vi "ABR3-Averager.vi"(0 "Runtime":T27={"Ceiling"=0.0, "Threshold"=0.0, "Crossed?"=FALSE, "Step"=0, "Stop"=0, "Avgs"=0, "Level"=0.0, "AI Npts"=0, "Doubled?"=FALSE, "Gain"=0.0, "NWindowPts"=0, "dt"=0.0, "Cal"=path "", "Freq"=0.0, "AO Channels"=[], "AltPol"=FALSE, "AO Npts"=0, "AO Fs"=0.0, "Start"=0, "Stop max"=0, "Ear"=enum."Right", "Waveform"=enum."TONE PIP", "RepRate"=0.0, "CAP or ABR"=1, "LMasker"=0.0, "SeqVar"=enum."Signal Level", "Reps/buffer"=0, "Avg Mode"=enum."Neural/CM", "Wav"=path "", "Order"=enum."Sequential", "Levels"=[], "ControlVal"=0.0, "innerIndex"=0, "indexStep"=0} {"CAP or ABR" items=["CAP", "ABR"]}, 2 "Abort":refnum<vi>, 7 "StimChans":T1 {"Filter"."Stages"."IIR Filter"."Forward Coefficients" format="%.4f"; "Filter"."Stages"."IIR Filter"."Reverse Coefficients" format="%.4f"}, 9 "Output Scaling":enum16{"Volts", "mV", "uV"}(ring)=enum."uV", 11 "error in (no error)":errorcluster, 12 "Remove DC Offset":bool=TRUE) -> (4 "Neural (uV)":dbl[](array[numeric])=[1.4395282511290837, 1.532755910405911, 1.474410329802132, 1.2597141561756957, 0.9001139821787747, 0.4235794582247189, -0.1276333716652575, -0.6998551074240021, -1.2340253166383555, -1.6719709249654355, -1.9620685245277936, -2.0664055181998617, -1.9647336236375028, -1.6568425026802076, -1.1650092311107514, -0.532397946197658, 0.18204236523367556, 0.906952954377487, 1.568756269865719, 2.0968412700840853, 2.432608440857153, 2.535322639805393, 2.3877606906196944, 1.9984937834608272, 1.4008932321747913, 0.6517150331153516, -0.17654328788016557, -1.0008408901491515, -1.7371580487858334, -2.3098045051007574, -2.65880868149595, -2.7463184287015, -2.5615615674647567, -2.121076834648578, -1.4686197069452032, -0.6693878326519646, 0.1969045084035855, 1.0449419706065644, 1.7920868586870562, 2.3650781681900184, 2.708422476925283, 2.788258951221298, 2.5965134974653075, 2.1522809221634867, 1.499118892634998, 0.7006198878547872, -0.1655836933809833, -1.014234830616595, -1.7625943927765395, -2.3380277004402488, -2.6840320769034283, -2.7664930928624387, -2.577696725613432, -2.1357488319848748, -1.4844911055883332, -0.6869176095510444, 0.17875347261089547, 1.0279345576657934, 1.7780792466594524, 2.355328107270133, 2.7038276454865047, 2.789379765791016, 2.60328656101914, 2.1640114189129878, 1.5144932790531567, 0.7183829551330373, -0.14731347632345962, -0.9972781324467478, -1.7485157781425051, -2.3281762074883967, -2.6794144228663423, -2.767570799346762, -2.5843785020013836, -2.1474007209849293, -1.4999111371554372, -0.7047973229346518, 0.1603615387991024, 1.0107597841892353, 1.7639270959139701, 2.3453802559937347, 2.6991542049437, 2.7904042207387056, 2.6098719770818493, 2.175698807779738, 1.5300274194957273, 0.7360268414650899, -0.128827718950226, -0.97999939173869, -1.7344067345971401, -2.3181269242110836, -2.6746496937413387, -2.768354355340884, -2.590961383132333, -2.159006966335281, -1.5152474886200955, -0.7225629269268649, 0.14208878618494694, 0.9936458695053323, 1.7493844364731472, 2.3354146545365095, 2.6944680855781407, 2.7912917435799787, 2.6162798887646694, 2.1871579771640977, 1.5453764489455355, 0.7535160460710334, -0.11053721586306206, -0.962852511425284, -1.7199756482361281, -2.308184143825026, -2.6697759261858742, -2.7692494856355405, -2.597356616772928, -2.1703317409173235, -1.5306421632430864, -0.7401205980371353, 0.12379574745708481, 0.9764888470355151, 1.7351688921529747, 2.3253704442717336, 2.6894371003402995, 2.791945974715928, 2.6226878005953473, 2.1984294994708335, 1.560659548702068, 0.7711371109548816, -0.09225432013500647, -0.9458070622432678, -1.705684029790087, -2.297977642892851, -2.6647373329909874, -2.7699873975748868, -2.603721421193753, -2.181846698979479, -1.5459100496436555, -0.75789888139616, 0.10526181069266684, 0.9592126436638952, 1.7207175213235073, 2.3148342936501165, 2.6843224344912207, 2.792615420540496, 2.628991745616928, 2.209772023817738, 1.575752465912369, 0.7890193603861616, -0.07390549445381299, -0.9283153177772733, -1.691212371809544, -2.2875175645807033, -2.6595694152244445, -2.770578234287441, -2.609946757906796, -2.193143580619579, -1.5610410047193342, -0.775284120672885, 0.08693073548743217, 0.9417944374520653, 1.7060962540767397, 2.304544113599402, 2.6792686273907975, 2.793145398476443, 2.6352703329820977, 2.220942115663773, 1.5908428477332726, 0.8064705291851398, -0.05570374342245042, -0.9110492571901601, -1.676634211761152, -2.2771462387137853, -2.6543583892194644, -2.77099917377202, -2.616113771792062, -2.204300994909238, -1.5763063561495347, -0.7928925079755119, 0.06860980337863325, 0.9246779881956217, 1.6914268075380636, 2.294053607483168, 2.6740778883452796, 2.7935206938641066, 2.6413714159532464, 2.232084314306749, 1.6060422681610205, 0.8241625963892981, -0.03717487820180634, -0.8937806611422894, -1.6619926577887165, -2.2666506600838408, -2.6490991835183375, -2.771371933418275, -2.6220931381771617, -2.215283440936453, -1.5912902371939535, -0.8106302198319645, 0.05024322743833475, 0.907150744453164, 1.676990652486208, 2.2835986025019612, 2.6686487861421813, 2.7937818791869247, 2.647264565187043, 2.243013508077417, 1.6209424678155986, 0.8417912696118693, -0.018957912612517995, -0.8762762387543624, -1.6472801025639217, -2.2559927920535903, -2.6437131889822236, -2.771732014155341, -2.627943179941323, -2.226303923886866, -1.60628172595746, -0.8280357460850919, 0.031891866119443904, 0.8898288983823229, 1.6621284879701426, 2.273057381400807, 2.662991463967972, 2.7940456002231904, 2.653058819196084, 2.253805770232825, 1.6358578824782266, 0.8590167556607577, -0.0005380855097547682, -0.8589315701916806, -1.6324483663924145, -2.2454338195540005, -2.63805333037468, -2.771828373804143, -2.633742506225171, -2.2371874752419902, -1.6212554647154789, -0.845656813087822, 0.013472039033399833, 0.8726896280383284, 1.6471598213917418, 2.2621789023862293, 2.657415286783958, 2.794157174537408, 2.6585893522697233, 2.2648110378220814, 1.650829084530336, 0.8768051829424925, 0.017838633505439176, -0.8413891118434587, -1.6174644842500803, -2.234560411108988, -2.6323605067511378, -2.7718765536431547, -2.639458151899738, -2.248114135072439, -1.6360364851212237, -0.8631434845611444, -0.00492496613723117, 0.8549062723626905, 1.6324700901986882, 2.251280137430886, 2.6516717483009025, 2.7940684222685657, 2.664284711061999, 2.275598228985624, 1.6655999609317433, 0.8940458841581485, 0.03615956559409267, -0.8238770830261509, -1.6026809285518098, -2.223684467145914, -2.6265130006914403, -2.7716102967650222, -2.644950649097256, -2.2585792839095884, -1.6507110034704318, -0.8803157208139684, -0.023197718633086662, 0.8375489263325268, 1.6173619569017978, 2.2404016589553764, 2.645727883422537, 2.7938047012037854, 2.669830459010278, 2.286111556607921, 1.6802770141117271, 0.9112536206390183, 0.054675751908509915, -0.8063447683355018, -1.5876716894773257, -2.2126056614032725, -2.6205310984515395, -2.771377004987947, -2.6503746803828574, -2.26918643648586, -1.6654844173387813, -0.8979088952371275, -0.04167840421967746, 0.8198315012253321, 1.6024161134418988, 2.229322854486931, 2.639796697528131, 2.7935866241444525, 2.675234203426622, 2.296594455191442, 1.6950199977826657, 0.9287935433005925, 0.07293075400881417, -0.7887389165905049, -1.5725052328839124, -2.2015420706085287, -2.614508623853641, -2.7710194600020954, -2.6556567081065747, -2.2796870867417764, -1.6801538649249124, -0.9152256709988795, -0.05998665753082091, 0.802261151042639, 1.5873079809104267, 2.218411411520159, 2.6337640806194615, 2.7930820040137405, 2.680465514967574, 2.307072282498074, 1.70971987368572, 0.9460393169109486, 0.09130747304302385, -0.7710519204811589, -1.5574199214201694, -2.1904429792523774, -2.6085013640321106, -2.770519911348151, -2.6609463432756186, -2.29005334112161, -1.6946305941277193, -0.9324156585420217, -0.07840394894946831, 0.7847846246058203, 1.572093346330642, 2.20700042102332, 2.6275083153116934, 2.7925469545091675, 2.685757685287872, 2.317400499277337, 1.7240393840276242, 0.9633129842890915, 0.10968419209879166, -0.753651466650922, -1.5422357152114121, -2.1789914153566126, -2.6022532053450385, -2.7699392177555886, -2.665908862976646, -2.300290271169476, -1.7091681822925784, -0.9498921884640046, -0.09663866502852804, 0.7669708410226813, 1.55699535766433, 2.1958100433093706, 2.6213565169854682, 2.7918318646607405, 2.690595951286384, 2.327591784368511, 1.7385769712468833, 0.9806018665855719, 0.12802794618370078, -0.7359061483634411, -1.5270160085834796, -2.1676793194380464, -2.5960050467862326, -2.769203841576933, -2.670929705707365, -2.3104764859072207, -1.7235891252756244, -0.9670162466031, -0.11484295192375675, 0.7493421688916414, 1.5416869002770077, 2.184388910315485, 2.614849709831871, 2.7910026647306077, 2.695581292511742, 2.3377298184180635, 1.7530892011204837, 0.9976042071355885, 0.14649088145417494, -0.7183129765330382, -1.511601047868935, -2.1561973268370647, -2.589450059108852, -2.768212351653958, -2.6758161521845514, -2.320769203572741, -1.7376753465564172, -0.9841326977485383, -0.13324249309905548, 0.7320000389875209, 1.526378443274855, 2.172851131977019, 2.608287115690693, 2.7900568189398456, 2.7003485568099435, 2.3478044583237763, 1.767177957231152, 1.014984377778882, 0.1648346356155949, -0.7006411960887469, -1.4962139810501114, -2.1447127987785337, -2.582753067945189, -2.76718028921617, -2.6804997364251566, -2.3305851954349137, -1.7520278244533696, -1.0014063669930806, -0.15151271010604112, 0.714077218032654, 1.510943198040489, 2.161211922902419, 2.6014988373813863, 2.7890627933674765, 2.7049180304571885, 2.3577624527603387, 1.7815025406516098, 1.032047577434772, 0.1830313152130599, -0.6827285177541538, -1.480864951204245, -2.133030480539171, -2.575929288016269, -2.7661456910403874, -2.6850666748634477, -2.3403682224641917, -1.7660962960808266, -1.0182641701842496, -0.17005425448429284, 0.6962938646504973, 1.4952518401973722, 2.149516927099661, 2.5947587389858833, 2.7878380118160977, 2.7093911444998424, 2.367395868027308, 1.7957307650661247, 1.0489358092347998, 0.20144860678364765, -0.6650212370259554, -1.4651786640447881, -2.1212391242885063, -2.5691460806573256, -2.7648575148560206, -2.6895372537110442, -2.350250145047671, -1.7802357697758513, -1.0355834839660625, -0.1882610774014398, 0.6784192237848757, 1.4798597038465398, 2.13772810790351, 2.5878386004844325, 2.786491512905318, 2.713983440269239, 2.3771966448057107, 1.8096546970626046, 1.0661891923214208, 0.21971375226454914, -0.6470933445595164, -1.4495988797039707, -2.109404660144406, -2.5622918716404395, -2.7635591955570358, -2.694017975789843, -2.360066137666051, -1.7942104185697303, -1.0523804293216747, -0.2065490450127634, 0.6605800839202034, 1.4642393484020582, 2.125820107628723, 2.581037643661518, 2.7851830506465243, 2.718418517778739, 2.386999957583907, 1.8236217375547858, 1.0830850320699636, 0.23812597242670458, -0.6294215650763136, -1.4339404868196217, -2.0975169450698448, -2.5552829802913215, -2.762141694617366, -2.6982704777527546, -2.3694611915644925, -1.808202818153744, -1.069230626194157, -0.22486490617253674, 0.6428804116000764, 1.4482741283453793, 2.1139400011792007, 2.5738537845377714, 2.783613403096724, 2.722622839463714, 2.3965015131897376, 1.8375456702847826, 1.0999960867726546, 0.25627193689684197, -0.6113973138242079, -1.418208556934832, -2.0855049773296264, -2.5479900818666787, -2.7605187955318686, -2.702451977990576, -2.3789576767500487, -1.8221445026495653, -1.0862608631352142, -0.2431351235786486, 0.6248358748193603, 1.4326968817766805, 2.101839282613086, 2.56670289062944, 2.7819702179752674, 2.7267155868816295, 2.4057063831215246, 1.851363100909952, 1.1170719669011222, 0.27440015106205384, -0.593423778195461, -1.4024791632205018, -2.073292683680086, -2.5407986147622528, -2.7587970010102, -2.7063367920534986, -2.388028151619793, -1.835832610156751, -1.1029538428928658, -0.2616411676260088, 0.6069206624947833, 1.4169167738274846, 2.08950527309283, 2.559318705298538, 2.780210386993262, 2.730519255576555, 2.4150177558892056, 1.8650714936261625, 1.133648300526371, 0.29293915993025077, -0.5757063555185494, -1.3867066617596802, -2.061095604988597, -2.533401749733742, -2.757019419340479, -2.710231749269889, -2.397451099724693, -1.8495384684521923, -1.1197812188493002, -0.27975416754395616, 0.5890384153766166, 1.4007968728445, 2.0774045552023517, 2.551987771452443, 2.7783694110848027, 2.734388854527701, 2.4244533819758685, 1.8788052444530907, 1.1506151431865264, 0.31097355081361083, -0.5577201414662862, -1.3708251224930792, -2.0489365632824286, -2.525982062894162, -2.7550288322114613, -2.7139390588641694, -2.406623006120719, -1.8632595417744564, -1.136639024418934, -0.2980674933467866, 0.5710369872817437, 1.3851942696638073, 2.064999544634335, 2.544524977320814, 2.7763281086137757, 2.738068270089232, 2.433569500401233, 1.892191594643508, 1.1673131944801958, 0.32944662987850254, -0.539815072249307, -1.3548421527325196, -2.0364985866595875, -2.5183747286105334, -2.7528379184684173, -2.7176210106849936, -2.415554013900312, -1.8766737868174372, -1.1531697158764533, -0.3163022104208217, 0.5531648836200865, 1.3692366588161557, 2.052647785705688, 2.5367097102202263, 2.77426651989102, 2.7416995059391827, 2.4423990761528023, 1.9056109102562346, 1.1839833526370318, 0.34755962981494204, -0.5217832147506022, -1.338732394775463, -2.023999751783519, -2.5104504222139727, -2.7506825056572644, -2.721054456174375, -2.424416555892335, -1.8901260688365098, -1.1699336986288993, -0.3344278895390942, 0.5350417389593082, 1.3529417907182757, 2.0401895245525083, 2.529061804623173, 2.772067999116759, 2.7450365913761954, 2.4512083659474833, 1.9190378335383393, 1.2006687257661814, 0.365713202171782, -0.5036828916702697, -1.3227266038327146, -2.0114578090763104, -2.5027771580438016, -2.748483984603527, -2.7245234025946865, -2.4334692813996686, -1.903461705622813, -1.1865404639345887, -0.3528020741843035, 0.5170656691051284, 1.3369486798092405, 2.0276729409547323, 2.521213572754994, 2.7697046526819635, 2.7485004658019165, 2.460121622798475, 1.9324799718506473, 1.2171512375589537, 0.38406456465418054, -0.4856687849437102, -1.3065788100683984, -1.9988550081260086, -2.4948655309081023, -2.746059779182957, -2.727895989452707, -2.442057959828062, -1.9164702278679644, -1.2030914426382415, -0.37094296818746797, 0.49907945634375267, 1.3208211733750277, 2.014940816812523, 2.5132715172726376, 2.76717901640693, 2.751888266947193, 2.468766087491162, 1.9457091054933713, 1.2335602123332297, 0.40214713571509625, -0.4676597499372556, -1.2902712630602917, -1.985978343860765, -2.4868550085978316, -2.743544285699133, -2.731103750647599, -2.4506998897994006, -1.9297551499079513, -1.219604385136538, -0.38908386233475983, 0.48082191641692823, 1.304569414505728, 2.002041331921324, 2.505131671278596, 2.7645316627102106, 2.7550148828155105, 2.477446053212338, 1.958712555602921, 1.2502278361276218, 0.4204579261486709, -0.44944531777965124, -1.2741209342720257, -1.9731549312156869, -2.478715161777337, -2.7408943959175667, -2.734202473365503, -2.459235317300394, -1.9430705016025347, -1.2360082898295168, -0.4072678647114303, 0.4628382397472022, 1.288360764108287, 1.989233135263758, 2.4968777155193824, 2.761775270529009, 2.7580121739827734, 2.485826797431994, 1.97198226235536, 1.2663223759828894, 0.43853542594029116, -0.43136021003728786, -1.2578260668801813, -1.960260517237996, -2.4704257042637585, -2.7379883923770554, -2.737154120869973, -2.467550132340703, -1.9560105590457155, -1.2523589436955342, -0.4252895780008659, 0.44466438052441326, 1.2718326068925097, 1.9761840403993531, 2.4885045784086737, 2.759072129737366, 2.760989178932014, 2.494022430080994, 1.9849907847186021, 1.2828632119346168, 0.4567244997294825, -0.4132472089942173, -1.2413613031742499, -1.947297637710777, -2.4619130985201534, -2.7350925320090744, -2.739849654637991, -2.476001879577561, -1.9688136850221156, -1.2686107028535771, -0.4434634376195193, 0.4264119125985013, 1.2554895613448314, 1.9632008760101387, 2.48018215700205, 2.7561585192983045, 2.763661890395179, 2.502398103099653, 1.9977736235210932, 1.2992569735137212, 0.4749059663618254, -0.395189995035824, -1.2250740438404228, -1.934329686984774, -2.453550103807855, -2.7322296367830616, -2.7425781536119915, -2.4840910107416825, -1.9817917797900413, -1.284875141230547, -0.4615840462493072, 0.4082659471272895, 1.2391414446079814, 1.9500833159444133, 2.4717202680398254, 2.7529735805129256, 2.7663067082870416, 2.510558235239559, 2.0106705725154517, 1.3153160136362303, 0.4930316462238931, -0.3771048877654994, -1.208616888188332, -1.920923047663721, -2.4450400342361003, -2.7290878058482697, -2.745157041573262, -2.492147177009889, -1.9945162974540873, -1.301152258848653, -0.47960068850441295, 0.39000080063122333, 1.2226335746387296, 1.9368009309343408, 2.463002265760695, 2.7496821389891775, 2.768870381247518, 2.518581435549004, 2.02342551848756, 1.3316032735468908, 0.511101539322759, -0.3587104167783139, -1.1919213704095126, -1.9077015202389411, -2.4362789228363164, -2.7257405767933123, -2.747662391940525, -2.500122198520436, -2.0072002430902764, -1.317371054098585, -0.4977187617199302, 0.3719283727317753, 1.2061890992963278, 1.92351347472132, 2.4542969425528365, 2.7464591635474354, 2.7712387992446943, 2.5263916307111822, 2.035972531296324, 1.3478296753155836, 0.5291131098931647, -0.3406329171012239, -1.175489573194469, -1.8944647785399493, -2.4275330263440256, -2.722355311077759, -2.7500155955379855, -2.5078842148977607, -2.01982840201712, -1.3333464156500179, -0.5157607620370909, 0.3536733695635592, 1.1895113333591902, 1.9102589839359723, 2.4453329702870823, 2.7429597881868357, 2.773505786060023, 2.5340978591650125, 2.048481507809941, 1.363881109223582, 0.5471196090969712, -0.3223271983176138, -1.1588726650470516, -1.8813041104226378, -2.418487908311925, -2.718848327958181, -2.7522267955200954, -2.5158668441185466, -2.03249966948883, -1.3495094246851844, -0.5338433348609879, 0.3353143999708917, 1.172732136945969, 1.8967027364091325, 2.43645267889724, 2.739242335856683, 2.775711914191574, 2.5420323077444715, 2.0609473765130346, 1.3797905402927073, 0.5651844311816042, -0.30416601851249997, -1.1420655744232873, -1.8675982512369118, -2.409445326266602, -2.7151866623603533, -2.754473496425215, -2.523481785659771, -2.044747462863247, -1.3654847869969653, -0.5517712259384716, 0.3171075766438307, 1.1561735529387842, 1.883128738844377, 2.427422776844838, 2.7356897092249115, 2.7778723983060822, 2.5494621367288666, 2.0732179908859454, 1.3958064741286889, 0.5830463918891033, -0.28589833651752683, -1.125397951564641, -1.8541383625066221, -2.40048388934014, -2.7115021747773245, -2.7564869055888566, -2.5309623311651763, -2.0569343979867307, -1.3814474708374418, -0.5697295464547676, 0.29879425111070773, 1.1393233556203597, 1.8696029213461443, 2.4182584788446406, 2.731888576306216, 2.779789447598124, 2.5569274667466364, 2.085415068122787, 1.4116601189541702, 0.6010604989617646, -0.26755965309759877, -1.1084691446454, -1.8404958984414477, -2.391294232607866, -2.7076604688784283, -2.7583912762301237, -2.538356660340975, -2.069311516582715, -1.3972351868021582, -0.5875915079333405, 0.28062039298224223, 1.1225010521159988, 1.856039067605407, 2.4088583537645163, 2.7278287939194765, 2.781622816185109, 2.56428883002743, 2.097749077525349, 1.4274503698659096, 0.6189097812081693, -0.24937311594237316, -1.091781236314106, -1.8267951119573107, -2.3819143928813644, -2.703620972281197, -2.760181536797, -2.5454390889296374, -2.0813868782604774, -1.4129544373101186, -0.6053063949823206, 0.2624008910962351, 1.1056609985605057, 1.8420137034257023, 2.39957233892674, 2.723931301453807, 2.783253322407029, 2.5713078634310507, 2.109771186958021, 1.443126511416476, 0.636819922128619, -0.23102682542586872, -1.0748245366173617, -1.8127418532700716, -2.3725548395654346, -2.6995003307628203, -2.7616294670967103, -2.5528993486569473, -2.0934039174323193, -1.4287801906321023, -0.6233788257829277, 0.24387963275702965, 1.0857754847470877, 1.8183295781965265, 2.367766091419394, 2.681223712822552, 2.729535373267443, 2.510314800597094, 2.0495693551720833, 1.3966559576513389, 0.620880074203631, -0.19861208734554114, -0.9789115461709459, -1.6430833982317077, -2.128138969482868, -2.3907033965627424, -2.411093581531485, -2.1951569867251726, -1.7721872242646255, -1.191421823477356, -0.5169145371876932, 0.1811954183282487, 0.8320260192072704, 1.3735880428904998, 1.7568776462956084, 1.9517417122730605, 1.9484832424464051, 1.7574025513572042, 1.408447296149037, 0.9447283236692902, 0.419730160344384, -0.11159716737835836, -0.5955411458827827, -0.9874063775542169, -1.2546157802529583, -1.379784004482954, -1.3610801513550121, -1.2109675481519084, -0.9550093732829174, -0.627291518489845, -0.26658338192841746, 0.08874381043064897, 0.4034150203824767, 0.6498258847102212, 0.8098786040255699, 0.8766023213339516, 0.8521169252825707, 0.7488451579968964, 0.5856734491572843, 0.3851245162283366, 0.1722999400598037, -0.030586949941910264, -0.2034909073282034, -0.33348204757844413, -0.4118829650461492, -0.43841218486660727, -0.4169443608101003, -0.3569556643837709, -0.2693575135107263, -0.16766809566460772, -0.06467783047578858, 0.028854014681161364, 0.10485101608964346, 0.15798552308759484, 0.18696429320988187, 0.1926114511761961, 0.17884729607034774, 0.1507180086533576, 0.11386567543666899, 0.07446996588255672, 0.037034405949865054, 0.005588332752696505, -0.018004463411863306, -0.03256231411188295, -0.0387064827707768, -0.037732747415657235, -0.03162407952533104, -0.0224623455792114, -0.01218994475038231, -0.002381589680865408, 0.005978841201505198, 0.012041865234115462, 0.01583284010978839, 0.017579985052400333, 0.017714380817214773, 0.01692575661235741, 0.015518404735495985, 0.014085695167122504, 0.012924312897508946, 0.01187450447036647, 0.011341992949343146, 0.011128988340931728, 0.010905840655928301, 0.010931198347405932, 0.011080808727124046, 0.011068129881385325, 0.011098559111158375, 0.011073201419680913, 0.0111061664186016, 0.01112898834093141, 0.011134059879227318, 0.01113152411007946, 0.01110109488030622, 0.011108702187749387, 0.0111010948803062, 0.011101094880306198, 0.011093487572863183, 0.011141667186670394, 0.011113773726045204, 0.011128988340931543, 0.01111630949519282, 0.011096023342010609, 0.011116309495192893, 0.011151810263261631, 0.011088416034567443, 0.011052915266498896, 0.011101094880306087, 0.011078272957976618, 0.011136595648374877, 0.011161953339852548, 0.011144202955818366, 0.011078272957976353, 0.011149274494113844, 0.011116309495192633, 0.011131524110079437, 0.011116309495192746, 0.011096023342010588, 0.011060522573941708, 0.011123916802636231, 0.011172096416443577, 0.011085880265419842, 0.011113773726045183, 0.011149274494113596, 0.011156881801556922, 0.011083344496272, 0.011136595648374917, 0.01113152411007942, 0.011098559111158392, 0.011131524110079718, 0.011139131417522815, 0.01109602334201091, 0.011101094880306387, 0.011098559111158413, 0.011118845264340491, 0.011146738724965926, 0.011106166418601711, 0.01108588026541958, 0.01112138103348841, 0.011169560647295847, 0.011136595648374976, 0.011121381033488597, 0.011134059879227056, 0.011156881801556844, 0.011101094880306481, 0.011106166418601546, 0.011098559111158526, 0.011080808727124122, 0.011134059879226929, 0.011090951803715264, 0.01110363064945423, 0.011111237956897118, 0.011123916802636193, 0.011085880265419469, 0.011144202955818068, 0.011106166418601526, 0.011149274494113806, 0.011083344496271928, 0.011108702187749538, 0.011174632185591364, 0.01113152411007914, 0.011126452571783397, 0.011134059879227469, 0.011131524110079232, 0.011156881801556712, 0.011101094880306086, 0.011103630649453947, 0.01112138103348818, 0.011149274494113865, 0.011096023342010722, 0.011154346032409002, 0.011108702187749387, 0.0111416671866706, 0.011096023342010592, 0.011172096416443424, 0.01108588026541975, 0.011108702187749725, 0.011146738724965796, 0.011174632185591418, 0.011090951803715226, 0.011103630649453853, 0.011085880265419637, 0.011128988340931522, 0.011113773726044884, 0.011083344496271814, 0.011116309495192572, 0.011156881801556882, 0.011131524110079158, 0.011106166418601847, 0.011134059879227113, 0.011111237956897379, 0.011141667186670602, 0.011070665650533561, 0.01113913141752263, 0.01115688180155677, 0.011159417570704705, 0.011088416034567308, 0.011111237956897476, 0.011128988340931633, 0.011156881801557161, 0.011057986804794747, 0.011111237956897268, 0.011113773726045037, 0.011146738724965927, 0.01112898834093173, 0.01111630949519295, 0.011146738724965927, 0.011126452571783942, 0.011085880265419939, 0.011075737188828642, 0.011123916802636025, 0.011093487572863069, 0.011078272957976221, 0.011113773726044978, 0.011108702187749502, 0.011123916802635837, 0.01106559411223724, 0.011123916802636214, 0.011093487572862956, 0.011141667186670262, 0.011073201419681085, 0.011136595648374749, 0.011108702187749687, 0.0111568818015569, 0.01108334449627153, 0.011136595648374955, 0.011075737188828552, 0.01112898834093192, 0.01112391680263614, 0.011134059879227168, 0.011098559111158281, 0.011103630649454044, 0.011131524110079682, 0.011070665650533261, 0.011134059879226983, 0.011134059879227207, 0.011103630649454117, 0.01112645257178387, 0.011085880265419769, 0.011123916802636065, 0.011144202955818368, 0.011128988340931543, 0.011088416034567476, 0.01113152411007929, 0.011108702187749649, 0.01112645257178398, 0.011098559111158226, 0.011111237956897302, 0.011121381033488201, 0.011154346032409414, 0.011073201419681065, 0.01113913141752259, 0.011098559111158564, 0.011111237956897174, 0.011174632185591045, 0.011121381033488297, 0.01108334449627164, 0.011111237956897436, 0.011121381033488427, 0.011128988340931558, 0.011101094880306351, 0.011090951803715358, 0.011146738724965966, 0.011136595648374785, 0.011164489109000314, 0.011085880265419675, 0.01114927449411377, 0.011131524110079645, 0.011187311031329954, 0.011060522573942137, 0.011136595648374954, 0.011078272957976204, 0.011139131417522534, 0.011111237956897321, 0.011136595648374936, 0.011096023342010609, 0.011126452571783962, 0.01113405987922713, 0.01112138103348858, 0.011123916802636176, 0.011146738724965665, 0.01114673872496585, 0.011085880265419316, 0.011131524110079513, 0.011131524110079265, 0.01108080872712427, 0.011126452571784037, 0.011093487572862862, 0.011101094880306236, 0.01115434603240915, 0.011113773726045316, 0.011085880265419524, 0.011068129881385532, 0.011073201419680876, 0.011134059879226907, 0.011070665650533013, 0.011136595648375104, 0.011080808727124386, 0.011164489109000409, 0.011101094880306351, 0.011088416034567741, 0.011101094880306594, 0.011083344496271796, 0.011121381033488297, 0.011164489109000426, 0.011118845264340755, 0.011116309495192784, 0.011151810263261367, 0.011116309495192952, 0.011159417570704743, 0.011113773726045089, 0.011131524110079212, 0.011111237956897476, 0.011128988340931786, 0.011113773726044846, 0.011151810263261406, 0.01114166718667013, 0.011134059879226941, 0.011080808727124197, 0.011131524110079479, 0.011088416034567219, 0.011156881801556844, 0.011078272957976525, 0.011136595648374749, 0.01109095180371519, 0.011174632185591043, 0.011098559111158243, 0.011090951803715263, 0.011121381033487974, 0.011113773726045146, 0.011116309495192836, 0.011151810263261312, 0.011035164882464619, 0.011136595648374877, 0.011101094880306184, 0.011068129881385383, 0.011093487572862937, 0.011093487572863069, 0.011090951803715322, 0.011159417570704818, 0.011154346032409059, 0.011161953339852359, 0.01112898834093173, 0.011057986804794294, 0.011083344496271812, 0.011106166418601921, 0.011093487572862916, 0.011141667186670264, 0.011126452571783905, 0.0110605225739421, 0.011126452571784112, 0.011139131417522534, 0.011101094880306216, 0.011113773726044995, 0.01111884526434055, 0.011111237956897117, 0.011083344496272095, 0.011073201419680894, 0.01114420295581794, 0.011121381033488505, 0.011098559111158526, 0.01108841603456761, 0.011090951803715453, 0.011144202955818179, 0.011134059879227075, 0.01109855911115849, 0.011103630649454063, 0.011136595648374785, 0.011128988340931635, 0.011113773726044772, 0.01109855911115849, 0.0111847752621823, 0.011090951803715152, 0.011134059879227337, 0.011146738724966004, 0.011103630649454023, 0.011139131417522685, 0.011116309495192876, 0.0111340598792273, 0.011090951803715094, 0.0111112379568974, 0.01108588026541956, 0.011101094880306275, 0.011080808727124311, 0.011078272957976299, 0.011090951803715339, 0.011108702187749593, 0.011116309495192989, 0.011134059879227338, 0.011118845264340586, 0.011113773726045223, 0.01109855911115849, 0.011101094880306145, 0.011121381033488446, 0.01114420295581833, 0.011096023342010817, 0.01109348757286305, 0.011118845264340453, 0.011088416034567497, 0.011134059879227057, 0.011136595648374822, 0.011144202955818236, 0.011108702187749425, 0.011134059879227262, 0.011126452571783832, 0.011136595648375087, 0.011085880265419373, 0.011050379497351315, 0.011083344496271927, 0.011156881801556993, 0.011118845264340548, 0.011123916802636177, 0.011121381033488484, 0.011088416034567422, 0.011101094880306164, 0.011136595648375104, 0.011126452571783792, 0.011096023342010609, 0.011149274494113695, 0.011098559111158545, 0.011065594112237538, 0.011106166418601827, 0.011108702187749576, 0.011136595648375049, 0.01106559411223739, 0.01115181026326148, 0.011161953339852922, 0.011096023342010852, 0.011057986804794334, 0.011118845264340286, 0.011096023342010836, 0.011118845264340848, 0.011101094880306332, 0.011113773726045204, 0.011136595648374823, 0.011164489109000164, 0.011103630649453855, 0.011108702187749668, 0.011103630649453532, 0.011085880265419599, 0.011139131417522964, 0.011085880265419786, 0.011088416034567554, 0.01113659564837484, 0.011134059879227151, 0.011060522573941897, 0.011123916802635856, 0.011106166418601716, 0.011118845264340625, 0.01108588026541973, 0.011108702187749465, 0.011042772189907844, 0.011161953339852699, 0.01106559411223771, 0.011098559111158528, 0.011096023342010968, 0.011149274494113844, 0.01110109488030635, 0.011111237956897453, 0.011159417570704837, 0.011090951803715263, 0.011078272957976676, 0.011080808727124006, 0.011149274494113546, 0.011123916802636195, 0.011083344496272058, 0.011118845264340567, 0.01111377372604486, 0.01115434603240902, 0.011113773726045297, 0.011121381033488467, 0.011090951803715058, 0.01111123795689697, 0.011093487572863011, 0.01115688180155739, 0.011118845264340756, 0.011090951803715058, 0.011113773726045204, 0.011057986804794107, 0.011113773726044808, 0.01111123795689755, 0.01111377372604511, 0.011098559111158677, 0.011113773726045183, 0.011088416034567197, 0.01108080872712414, 0.01109095180371515, 0.011151810263261253, 0.011111237956897342, 0.011116309495192838, 0.011103630649453853, 0.011121381033488389, 0.011118845264340737, 0.011111237956897325, 0.011068129881385457, 0.01108588026541975, 0.011103630649454065, 0.011088416034567271, 0.011098559111158188, 0.01111377372604509, 0.011139131417522347, 0.01111123795689721, 0.01115434603240932, 0.01107066565053273, 0.01113913141752272, 0.011116309495192819, 0.011164489109000107, 0.011103630649454023, 0.011093487572862843, 0.011123916802635988, 0.01109855911115849, 0.011164489109000053, 0.011116309495192912, 0.01111884526434051, 0.011123916802635763, 0.011090951803715113, 0.011136595648374839, 0.011088416034567667, 0.011085880265419654, 0.011108702187749576, 0.011151810263261537, 0.011154346032408948, 0.011088416034567554, 0.011055451035646395, 0.011118845264340399, 0.011131524110079309, 0.01110363064945404, 0.011090951803715134, 0.011093487572862784, 0.011101094880306124, 0.011151810263261366, 0.011108702187749349, 0.011182239493034738, 0.011141667186670133, 0.011151810263261572, 0.011113773726045146, 0.011144202955818328, 0.011088416034567401, 0.011106166418601394, 0.01112645257178385, 0.011154346032409135, 0.011101094880306387, 0.0110782729579762, 0.011085880265419805, 0.011121381033488354, 0.011101094880306276, 0.011083344496271928, 0.011131524110079309, 0.011088416034567687, 0.011121381033488316, 0.011113773726045259, 0.011118845264340567, 0.011123916802636288, 0.0110985591111583, 0.011088416034567573, 0.011083344496272114, 0.01109348757286303, 0.011131524110079496, 0.011063058343089962, 0.011141667186670449, 0.011131524110079422, 0.011106166418601808, 0.011108702187749444, 0.011093487572862973, 0.011139131417522796, 0.011144202955818062, 0.01113405987922732, 0.011128988340931673, 0.011078272957976223, 0.011126452571784, 0.011154346032409286, 0.011106166418601753, 0.011108702187749687, 0.011126452571784016, 0.011113773726045316, 0.011106166418601677, 0.011070665650533166, 0.011106166418601753, 0.011078272957976353, 0.011128988340931524, 0.011060522573942142, 0.011151810263261498, 0.011093487572863388, 0.01108588026541958, 0.01107320141968099, 0.011164489109000182, 0.011096023342010741, 0.011134059879227132, 0.011085880265419542, 0.011121381033488448, 0.01113405987922747, 0.011106166418601788, 0.011118845264340304, 0.011128988340931673, 0.01109095180371536, 0.011093487572863181, 0.011111237956897474, 0.011139131417522477, 0.01113405987922732, 0.011088416034567516, 0.01111630949519265, 0.011111237956897248, 0.011139131417522702, 0.011088416034567573, 0.011096023342010743, 0.01113913141752276, 0.011093487572862975, 0.011222811799398704, 0.011118845264340718, 0.011151810263261461, 0.01106052257394206, 0.011126452571783903, 0.011113773726044995, 0.011083344496271588, 0.011116309495192838, 0.011118845264340382, 0.011139131417522664, 0.011134059879226997, 0.011101094880306124, 0.011113773726045016, 0.01108080872712401, 0.011106166418601808, 0.0111315241100791, 0.01109095180371515, 0.01110109488030633, 0.01106052257394212, 0.011098559111158528, 0.011068129881385365, 0.0111112379568974, 0.011134059879227247, 0.011136595648375104, 0.011101094880306313, 0.011088416034567271, 0.011090951803715192, 0.011136595648374917, 0.011113773726045037, 0.011090951803715223, 0.011090951803715209, 0.01116956064729579, 0.011098559111158509, 0.011126452571784035, 0.011172096416443558, 0.011123916802636233, 0.011093487572862862, 0.011126452571783981, 0.011111237956897453, 0.011078272957976318, 0.011078272957976637, 0.011136595648374745, 0.011111237956897547, 0.011128988340931692, 0.011144202955818272, 0.011098559111158564, 0.011073201419681102, 0.011141667186670283, 0.011101094880306145, 0.011128988340931355, 0.011131524110079326, 0.011128988340931449, 0.011123916802636157, 0.011093487572863239, 0.01109095180371513, 0.011123916802636288, 0.011128988340931617, 0.011065594112237521, 0.011121381033488299, 0.011073201419680722, 0.01111884526434055, 0.011156881801556901, 0.011131524110079534, 0.01108588026541958, 0.011098559111158472, 0.011116309495192553, 0.011118845264340716, 0.01112645257178398, 0.01114673872496621, 0.011134059879227207, 0.01111123795689736, 0.01119745410792087, 0.011159417570704684, 0.011093487572863011, 0.011118845264340418, 0.0111112379568971, 0.01113659564837441, 0.011167024878148192, 0.01108080872712429, 0.01112391680263631, 0.011085880265419654, 0.011128988340931427, 0.011136595648374954, 0.011108702187749595, 0.011149274494113787, 0.011073201419680953, 0.011113773726044883, 0.011123916802636327, 0.011103630649453928, 0.011149274494113525, 0.011098559111158677, 0.01109602334201078, 0.011167024878147988, 0.011123916802636347, 0.011080808727124308, 0.011156881801557201, 0.011042772189907749, 0.01112138103348824, 0.011096023342010871, 0.011098559111158791, 0.01112645257178385, 0.011118845264340678, 0.011045307959055629, 0.011121381033488446, 0.011121381033488014, 0.011141667186670338, 0.01106812988138521, 0.011090951803715209, 0.011101094880306108, 0.011116309495193063, 0.011128988340931765, 0.011080808727124141, 0.011134059879227281, 0.011121381033488482, 0.011106166418601753, 0.011111237956897436, 0.011136595648374954, 0.011111237956897361, 0.011118845264340345, 0.011144202955818217, 0.01110363064945408, 0.011123916802636177, 0.011063058343089675, 0.011093487572863181, 0.01108334449627172, 0.01112645257178398, 0.011113773726045184, 0.011113773726044938, 0.011121381033488429, 0.011149274494113712, 0.011088416034567759, 0.011144202955817953, 0.011106166418601845, 0.011164489109000314, 0.011037700651612064, 0.011106166418601881, 0.011093487572863048, 0.011085880265419689, 0.011118845264340621, 0.011101094880306351, 0.011131524110079345, 0.01109095180371502, 0.011106166418601978, 0.011136595648374764, 0.011103630649453985, 0.011123916802636327, 0.01114927449411336, 0.011090951803714947], 6 "microphonic (uV)":dbl[](array[numeric]), 8 "StimChans out":T1 {"Filter"."Stages"."IIR Filter"."Forward Coefficients" format="%.4f"; "Filter"."Stages"."IIR Filter"."Reverse Coefficients" format="%.4f"}, 10 "Averaging data":cluster{i32, i32}, 15 "error out":errorcluster)   [LabVIEW 2020]
uses:
  TypeDefs/ABR3-Runtime Data.ctl
  epl-vi-lib/Utility VIs/Type Defs/Left-Right ring.ctl
  TypeDefs/ABR-Waveform Enum.ctl
  TypeDefs/ABR3-Seq Var Enum.ctl
  epl-vi-lib/Signal Synthesis VIs/Controls/Multichannel (Full)/Data.ctl
  epl-vi-lib/Signal Synthesis VIs/Controls/Stimulus Channel (Full)/Full Stimulus Channel Data.ctl
  epl-vi-lib/Signal Synthesis VIs/Controls/Waveform XCtl/Waveform Data.ctl
  epl-vi-lib/Signal Synthesis VIs/Controls/Waveform XCtl/Waveform Enum.ctl
  epl-vi-lib/Signal Synthesis VIs/Waveform VIs/Tone VIs/Tone Params.ctl
  epl-vi-lib/Signal Synthesis VIs/Waveform VIs/Pulse Train VIs/Pulse Train Params.ctl
  epl-vi-lib/Signal Synthesis VIs/Waveform VIs/Pulse Train VIs/Pulse Polarity.ctl
  epl-vi-lib/Signal Synthesis VIs/Waveform VIs/Pulse Train VIs/PT-Continuous State.ctl
  epl-vi-lib/Signal Synthesis VIs/Waveform VIs/Noise VIs/Noise Params.ctl
  epl-vi-lib/Signal Synthesis VIs/Waveform VIs/File VIs/StimFile-Params.ctl
  epl-vi-lib/Signal Synthesis VIs/Waveform VIs/FM Sweep VIs/FM Sweep Params.ctl
  epl-vi-lib/Signal Synthesis VIs/Waveform VIs/Chirp Train VIs/Chirp Train.ctl
  epl-vi-lib/Signal Synthesis VIs/Waveform VIs/Chirp Train VIs/Chirp Train Params.ctl
  epl-vi-lib/Signal Synthesis VIs/Waveform VIs/Complex Tone VIs/CT-Params.ctl
  epl-vi-lib/Signal Synthesis VIs/Waveform VIs/Complex Tone VIs/CT-Phase Enum.ctl
  epl-vi-lib/Signal Synthesis VIs/Waveform VIs/Complex Tone VIs/CT-Runtime Data.ctl
  epl-vi-lib/Signal Synthesis VIs/Waveform VIs/Moving Ripple VIs/Moving Ripple.ctl
  epl-vi-lib/Signal Synthesis VIs/Waveform VIs/Moving Ripple VIs/Moving Ripple.Params.ctl
  epl-vi-lib/Signal Synthesis VIs/Waveform VIs/Moving Ripple VIs/Moving Ripple.Data.ctl
  epl-vi-lib/Signal Synthesis VIs/Controls/Advanced Filter XCtl/Filter Data.ctl
  epl-vi-lib/Signal Synthesis VIs/Filter VIs/Filter-Bandwidth Units.ctl
  epl-vi-lib/Signal Synthesis VIs/Controls/Burst XCtl/Burst Data.ctl
  epl-vi-lib/Signal Synthesis VIs/Controls/Level XCtl/Level Data.ctl
  epl-vi-lib/Signal Synthesis VIs/Controls/Level XCtl/Level Units.ctl
  epl-vi-lib/Signal Synthesis VIs/Controls/Advanced Options XCtl/Advanced Stimulus Options.ctl
  epl-vi-lib/Signal Synthesis VIs/Modulation VIs/SAM VIs/SAM Params.ctl
  epl-vi-lib/PXI DAQ VIs/DAQ Engine VIs/PXI Globals.vi
  epl-vi-lib/Utility VIs/Conversion VIs/Create Waveform Cluster (2D).vi
  epl-vi-lib/Signal Synthesis VIs/Controls/Advanced Filter XCtl/Advanced Filter XCtl.xctl
  epl-vi-lib/Signal Synthesis VIs/Controls/Level XCtl/Level XCtl.xctl
  epl-vi-lib/Signal Synthesis VIs/Controls/Burst XCtl/Burst Control.xctl
  epl-vi-lib/Signal Synthesis VIs/Controls/Waveform XCtl/Waveform XCtl.xctl
  epl-vi-lib/Signal Synthesis VIs/Controls/Stimulus Channel (Full)/Stimulus Channel (Full).xctl
  epl-vi-lib/Signal Synthesis VIs/Controls/Multichannel (Full)/Multichannel (Full).xctl
  epl-vi-lib/Signal Synthesis VIs/Controls/Advanced Options XCtl/Advanced Stimulus Options.xctl
panel:
  out "Error":bool
  in  "Reject Override":bool
  in  "Rej Thresh µV":dbl=15.0
  out "Reject":bool
  out "Average":cluster{"offset":dbl, "dx":dbl, "Y":dbl[][]}(graph)
  out "#Aves":i32=120
  out "#Tries":i32=120
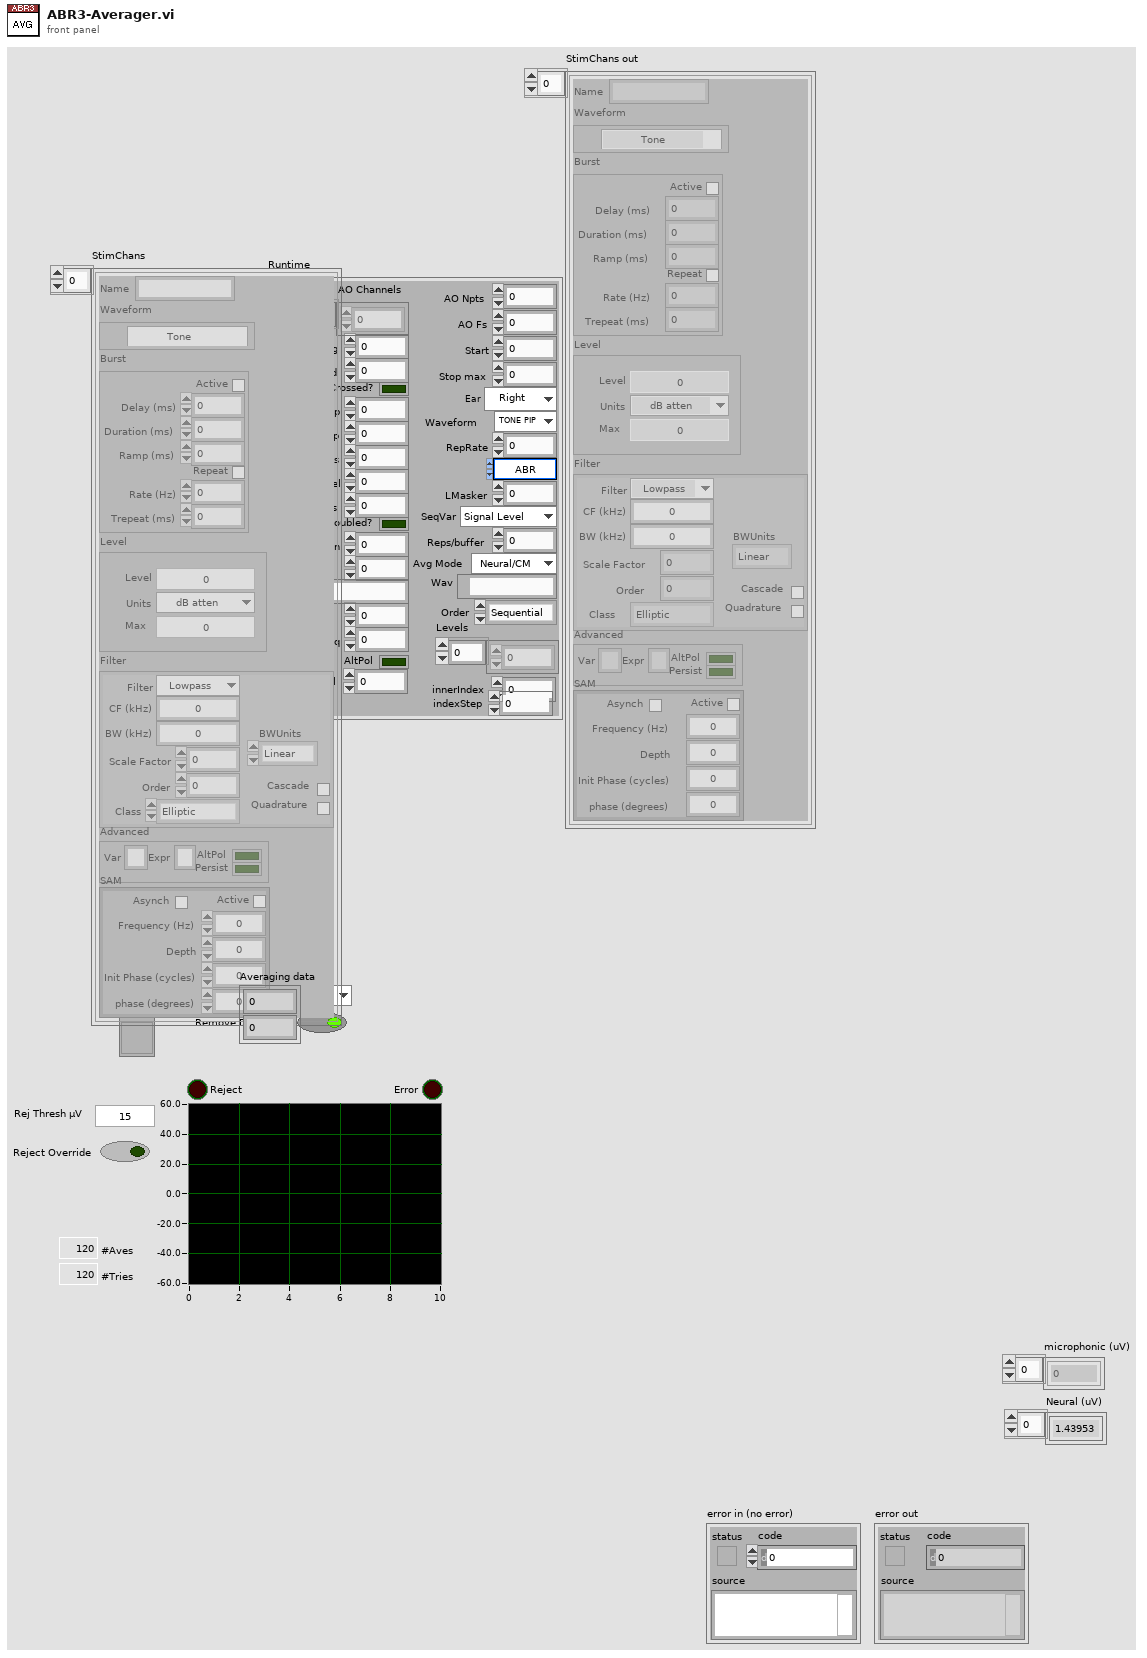
[diagram p1: front panel]
types:
  T1 = typedef "Multichannel (Full).xctl/Data.ctl" = T2[]
  T2 = typedef "Stimulus Channel (Full).xctl/Full Stimulus Channel Data.ctl" = cluster{"Waveform":T3, "Filter":T20, "Burst":T22, "Level":T23, "Name":string, "Advanced":T25, "SAM":T26}
  T3 = typedef "Waveform XCtl.xctl/Waveform Data.ctl" = cluster{"Type":T4, "Tone":T5, "Pulse Train":T6, "Noise":T9, "File":T10, "FMSweep":T11, "Chirp Train":T12, "Complex Tone":cluster{"Params":T14, "Data":T16}, "Moving Ripple":T17}
  T4 = typedef "Waveform Enum.ctl" = enum16{"OFF", "Tone", "Noise", "Pulse Train", "File", "FM Sweep", "Chirp Train", "Complex Tone", "FM Tone", "Moving Ripple"}
  T5 = typedef "Tone Params.ctl" = cluster{"Frequency (kHz)":dbl, "Last Freq":dbl, "Last Phase":dbl}
  T6 = typedef "Pulse Train Params.ctl" = cluster{"Pulse width (us)":dbl, "Pulse rate (Hz)":dbl, "Gap (ms)":dbl, "Polarity":T7, "PT State":T8, "Asynch":bool}
  T7 = typedef "Pulse Polarity.ctl" = enum16{"POS", "NEG", "POS-NEG", "NEG-POS"}
  T8 = typedef "PT-Continuous State.ctl" = cluster{"Template":dbl[], "Nperiod":i32, "Index":i32, "Pulse Rate (Hz)":dbl, "Phase (cycles)":dbl, "Noff":i32}
  T9 = typedef "Noise Params.ctl" = cluster{"InvFilt":bool, "Noise":dbl[], "CurPt":i32, "Aweight":bool, "Seed":i32, "afile":path}
  T10 = typedef "StimFile-Params.ctl" = cluster{"Filename":path, "Signal":dbl[], "Channel":i32, "stream":bool, "offset":i32, "nreps":i32, "loops":i32, "Randomize":bool, "order":i32[], "Seed":i32, "Tokens":i32}
  T11 = typedef "FM Sweep Params.ctl" = cluster{"Rate (oct/s)":dbl, "Fmin (Hz)":dbl, "Fmax (Hz)":dbl, "Ramp (ms)":dbl, "Linear":bool}
  T12 = typedef "Chirp Train.ctl" = cluster{"Params":T13, "Data":cluster{"WF":dbl[]}}
  T13 = typedef "Chirp Train Params.ctl" = cluster{"Fmin (kHz)":dbl, "Fmax (kHz)":dbl, "Compensate":bool, "Duration (ms)":dbl}
  T14 = typedef "CT-Params.ctl" = cluster{"F0 (Hz)":dbl, "Band":cluster{"Flow (Hz)":dbl, "Fhigh (Hz)":dbl}, "Phase":T15, "Min F0 (Hz)":dbl, "Max F0 (Hz)":dbl, "ContinRandPhase":bool, "Max peak factor":dbl, "Max mod depth":dbl, "MinHarmNum":i32, "MaxHarmNum":i32, "Level Mode":enum16{"per component", "overall rms"}, "% jitter":dbl}
  T15 = typedef "CT-Phase Enum.ctl" = enum16{"Cosine", "Random", "Alternating"}
  T16 = typedef "CT-Runtime Data.ctl" = cluster{"Ncomp":i32, "MinHarm":i32, "Phase":dbl[], "Amplitude":dbl[], "Npts/frame":i32, "Last F0":dbl, "Fmin":dbl, "Fmax":dbl, "Lslope":dbl, "randphase":bool, "overall rms":bool, "fmult":dbl[], "jittered":bool}
  T17 = typedef "Moving Ripple.ctl" = cluster{"Params":T18, "Data":T19}
  T18 = typedef "Moving Ripple.Params.ctl" = cluster{"Fmin":dbl, "Fmax":dbl, "Density":dbl, "Velocity":dbl, "Depth":dbl, "Phase":dbl, "Comp/oct":i32}
  T19 = typedef "Moving Ripple.Data.ctl" = cluster{"Freq":dbl[], "A":dbl[], "phase":dbl[], "Phase":dbl}
  T20 = typedef "Advanced Filter XCtl.xctl/Filter Data.ctl" = cluster{"Type":enum16{"Lowpass", "Highpass", "Bandpass", "Bandstop", "OFF"}, "CF (kHz)":dbl, "BW (kHz)":dbl, "Cascade":bool, "Quadrature":bool, "Scale Factor":dbl, "Stages":cluster{"IIR Filter":cluster{"filter structure":enum32{"IIR 2nd Order", "IIR 4th Order"}, "Reverse Coefficients":dbl[], "Forward Coefficients":dbl[]}, "State":dbl[]}[], "Class":enum16{"Elliptic", "Butterworth"}, "Order":i32, "BWUnits":T21}
  T21 = typedef "Filter-Bandwidth Units.ctl" = enum16{"Linear", "Octaves", "Min-Max"}
  T22 = typedef "Burst Control.xctl/Burst Data.ctl" = cluster{"Active":bool, "Delay (ms)":dbl, "Duration (ms)":dbl, "Ramp (ms)":dbl, "Rate (Hz)":dbl, "Trepeat (ms)":dbl, "Repeat":bool}
  T23 = typedef "Level XCtl.xctl/Level Data.ctl" = cluster{"Level":dbl, "Units":T24, "Max":dbl, "Multiplier":dbl, "Cal File":path, "Cal":cluster{"Freq (Hz)":dbl[], "Mag (dB SPL)":dbl[], "Phase (deg)":dbl[]}}
  T24 = typedef "Level Units.ctl" = enum16{"dB atten", "dB SPL", "dB re 1 Vrms", "dB V/Hz½", "mW", "dB HL", "Volts", "dB mW"}
  T25 = typedef "Advanced Stimulus Options.xctl/Advanced Stimulus Options.ctl" = cluster{"Rep Mask":string, "AltPol":bool, "Var":string, "Expr":string, "Persist":bool}
  T26 = typedef "SAM Params.ctl" = cluster{"Active":bool, "Frequency (Hz)":dbl, "Depth":dbl, "Init Phase (cycles)":dbl, "phase (degrees)":dbl, "Asynch":bool}
  T27 = typedef "ABR3-Runtime Data.ctl" = cluster{"Ceiling":dbl, "Threshold":dbl, "Crossed?":bool, "Step":i32, "Stop":i32, "Avgs":i32, "Level":dbl, "AI Npts":i32, "Doubled?":bool, "Gain":dbl, "NWindowPts":i32, "dt":dbl, "Cal":path, "Freq":dbl, "AO Channels":i32[], "AltPol":bool, "AO Npts":i32, "AO Fs":dbl, "Start":i32, "Stop max":i32, "Ear":T28, "Waveform":T29, "RepRate":dbl, "CAP or ABR":u16, "LMasker":dbl, "SeqVar":T30, "Reps/buffer":i32, "Avg Mode":enum16{"Neural/CM", "ANOW"}, "Wav":path, "Order":enum16{"Sequential", "Random"}, "Levels":dbl[], "ControlVal":dbl, "innerIndex":i32, "indexStep":i32}
  T28 = typedef "Left-Right ring.ctl" = enum16{"Right", "Left"}
  T29 = typedef "ABR-Waveform Enum.ctl" = enum16{"TONE PIP", "CLICK", "FILE", "CHIRP", "NOISE", "VERHULST"}
  T30 = typedef "ABR3-Seq Var Enum.ctl" = enum16{"Signal Level", "Masker Level"}
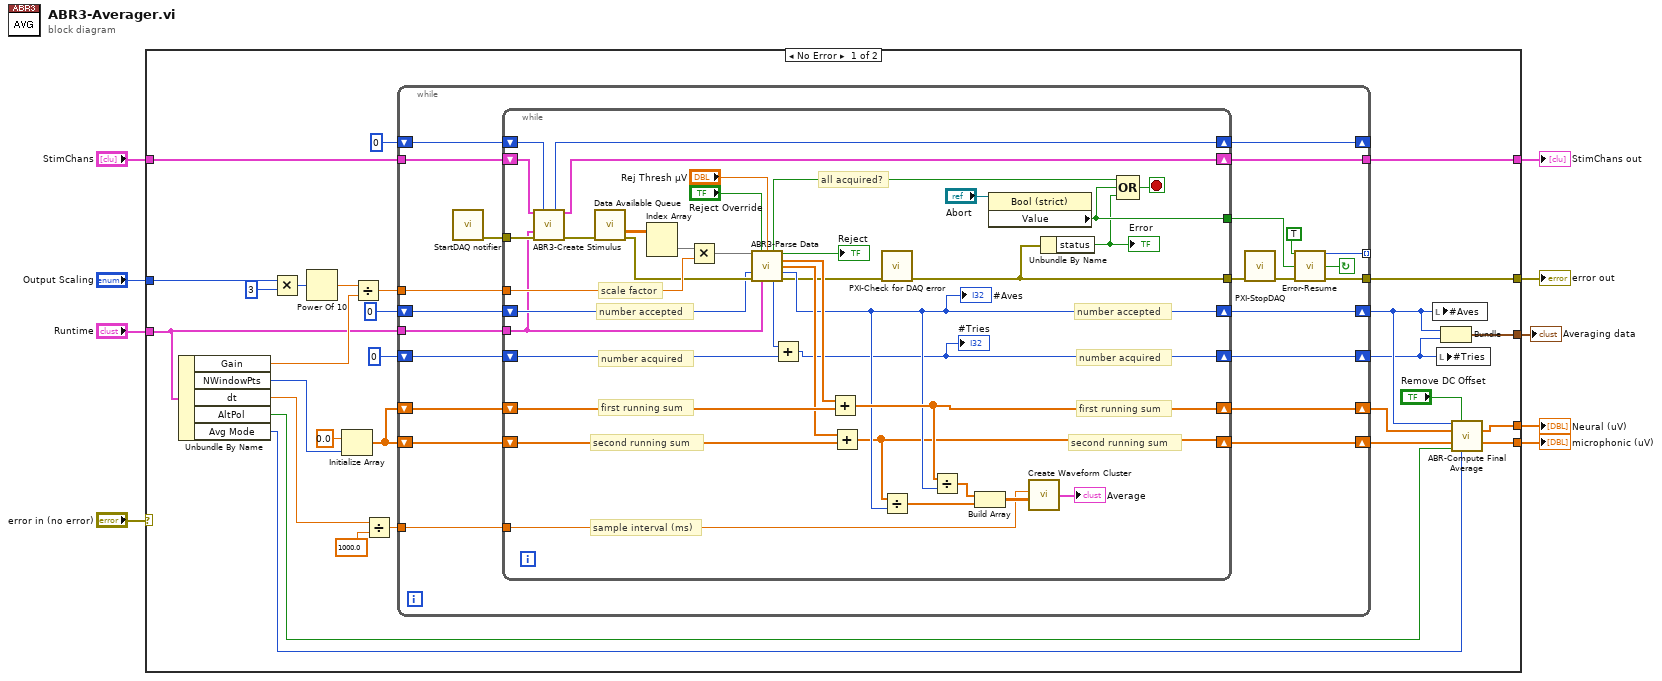
[diagram p0: block diagram]
diagram:
  n1 = case shown="No Error" "error in (no error)" {
    selector: "error in (no error)" -> [_ w100]
    tunnel: "Output Scaling" -> [w34 _]
    tunnel: [w28 _] -> w8
    tunnel: "Runtime" -> [w18 _]
    tunnel: "StimChans" -> [w25 _]
    tunnel: [w23 _] -> w5
    tunnel: [w22 _] -> w4
    tunnel: [w21 w100] -> w2
    tunnel: [w11 _] -> w1
    frame No Error {
      n2 = Unbundle By Name(w18) -> ("Gain"=w27:dbl, "NWindowPts"=w17:i32, "dt"=w26:dbl, "AltPol"=w24:bool, "Avg Mode"=w14:enum16{"Neural/CM", "ANOW"})
      n3 = Multiply(x=w34, y=3) -> (x*y=w31:i32)
      n4 = Power Of 10(x=w31) -> (10^x=w32:dbl)
      n5 = Initialize Array(0.0, w17) -> (w20:dbl[])
      n6 = Divide(x=w32, y=w27) -> (x/y=w37:dbl)
      n7 = Divide(x=w26, y=1000.0) -> (x/y=w29:dbl)
      n8 = while {
        tunnel: w37 -> [w61]
        tunnel: w29 -> [w57]
        tunnel: w25 -> [w54]
        tunnel: [w53] -> w22
        tunnel: [w49] -> w21
        tunnel: [w47] -> _ mode=indexing
        shift-right: [w58] -> w15
        shift-left: w20 -> [w45]
        shift-right: [w59] -> w35
        shift-left: w20 -> [w44]
        shift-right: [w55] -> w12
        shift-left: 0 -> [w43]
        shift-right: [w56] -> w13
        shift-left: 0 -> [w60]
        tunnel: w18 -> [w42]
        shift-right: [w39] -> _
        shift-left: 0 -> [w40]
        stop <- w48 continue-if-true
        n9 = call "StartDAQ notifier.vi"() -> ("error out"=w52:errorcluster)  [unwired: 7 in]
        n10 = while {
          shift-right: [w72] -> w59
          shift-left: w44 -> [w97]
          shift-right: [w65] -> w58
          shift-left: w45 -> [w99]
          tunnel: w61 -> [w92]
          shift-right: [w71] -> w56
          shift-left: w60 -> [w77]
          tunnel: w57 -> [w93]
          tunnel: [w89] -> w50
          shift-right: [w85] -> w53
          shift-left: w54 -> [w86]
          tunnel: w52 -> [w84]
          tunnel: [w83] -> w46
          shift-right: [w67] -> w55
          shift-left: w43 -> [w81]
          tunnel: w42 -> [w66]
          shift-right: [w63] -> w39
          shift-left: w40 -> [w64]
          stop <- w94 stop-if-true
          # "scale factor"
          # "all acquired?"
          # "number acquired"
          # "number acquired"
          # "number accepted"
          # "number accepted"
          # "second running sum"
          # "first running sum"
          # "sample interval (ms)"
          # "second running sum"
          # "first running sum"
          n11 = call "ABR3-Create Stimulus.vi"("StimChans"=w86, "Rep In"=w64, "Runtime"=w66, "error in (no error)"=w84) -> ("Rep Out"=w63:i32, "StimChans out"=w85:T2[], "error out"=w87:errorcluster)  [unwired: 9 in]
          n12 = call "Data Available Queue.vi"("error in (no error)"=w87) -> ("AI Waveforms"=w90:dbl[][], "error out"=w78:errorcluster)  [unwired: 10 in, 3 out]
          n13 = Index Array(array=w90) -> (element=w91:dbl[])  [unwired: 2 in]
          n14 = Multiply(x=w91, y=w92) -> (x*y=w62:dbl[])
          n15 = call "ABR3-Parse Data.vi"("Data"=w62, "Reject OverRide"="Reject Override", "Rej Thresh µV"="Rej Thresh µV", "Acquired In"=w77, "error in (no error)"=w78, "Runtime"=w66) -> ("Finished?"=w69:bool, "Any rejected?"=→"Reject":bool, "RunSum1"=w75:dbl[], "RunSum2"=w74:dbl[], "Acquired Out"=w71:i32, "Ntries"=w68:i32, "error out"=w70:errorcluster)  [unwired: 3 in]
          "#Aves" <- w71
          n16 = Add(x=w68, y=w81) -> (x+y=w67:i32)
          "#Tries" <- w67
          n17 = Add(x=w75, y=w97) -> (x+y=w72:dbl[])
          n18 = Add(x=w74, y=w99) -> (x+y=w65:dbl[])
          n19 = call "PXI-Check for DAQ error.vi"("error in (no error)"=w70) -> ("error out"=w89:errorcluster)  [unwired: 14 in]
          n20 = Divide(x=w65, y=w71) -> (x/y=w98:dbl[])
          n21 = Divide(x=w72, y=w71) -> (x/y=w96:dbl[])
          n22 = Build Array(w96, w98) -> (w95:dbl[][])
          n23 = property class="Bool (strict)"(reference="Abort") -> ("Value"=w83:bool)  [unwired: 1 in, 2 out]
          n24 = call-poly "Create Waveform Cluster.vi"("dx"=w93, "Array"=w95) -> ("waveform cluster"=→"Average":cluster{"offset":dbl, "dx":dbl, "Y":dbl[][]})  [unwired: 3 in]
          n25 = Unbundle By Name(w89) -> ("status"=w82:bool)
          "Error" <- w82
          n26 = Compound Arithmetic op=OR(w69, w83, w82) -> (w94:bool)
        }
        n27 = call "PXI-StopDAQ.vi"("error in (no error)"=w50) -> ("error out"=w51:errorcluster)  [unwired: 6 in]
        n28 = call "Error-Resume.vi"("Ignore local?"=TRUE, "Abort"=w46, "error in (no error)"=w51) -> ("code"=w47:i32, "Resume?"=w48:bool, "error out"=w49:errorcluster)  [unwired: 10 in]
      }
      n29 = local write "#Aves"(w13) -> ()
      n30 = local write "#Tries"(w12) -> ()
      n31 = Bundle(w13, w12) -> (w11:cluster{i32, i32})  [unwired: 1 in]
      n32 = call "ABR-Compute Final Average.vi"("#Avgs"=w13, "Remove DC Offset"="Remove DC Offset", "Running Sum 1"=w35, "Running Sum 2"=w15, "AltPol"=w24, "Avg Mode"=w14) -> ("Neural"=w23:dbl[], "Microphonic"=w28:dbl[])  [unwired: 8 in]
    }
    frame Error {
    }
  }
  "microphonic (uV)" <- w8
  "Neural (uV)" <- w5
  "StimChans out" <- w4
  "error out" <- w2
  "Averaging data" <- w1
